vi "get_length.vi"(8 "error in (no error)":errorcluster, 11 "SpaceVector in":refnum<class "SpaceVector.lvclass">) -> (0 "error out":errorcluster, 2 "length":dbl[unit], 3 "SpaceVector out":refnum<class "SpaceVector.lvclass">)   [LabVIEW 2010, in "SpaceVector.lvclass"]
uses:
  SpaceVector.lvclass
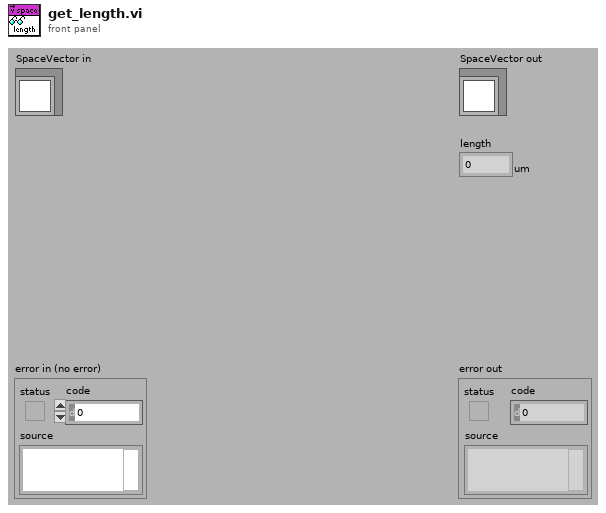
[diagram p1: front panel]
types:
  T1 = typedef "space_vector_array.ctl" = dbl[unit][]
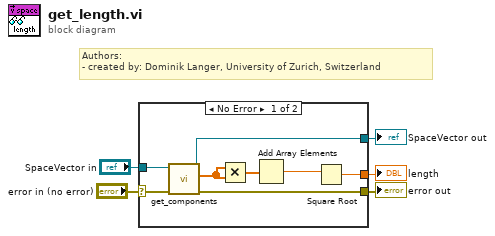
[diagram p0: block diagram]
diagram:
  # "Authors: \n- created by: Dominik Langer, University of Zurich, Switzerland"
  n1 = case shown="No Error" "error in (no error)" {
    selector: "error in (no error)" -> [w13 w15]
    tunnel: [w12 w15] -> w4
    tunnel: [w10 w14] -> w2
    tunnel: "SpaceVector in" -> [w11 w14]
    tunnel: [w6 _] -> w1
    frame No Error {
      n2 = call "get_components.vi"("error in (no error)"=w13, "SpaceVector in"=w11) -> ("error out"=w12:errorcluster, "x/y/z"=w9:T1, "SpaceVector out"=w10:refnum<class "SpaceVector.lvclass">)  [unwired: 4 in, 3 out]
      n3 = Multiply(x=w9, y=w9) -> (x*y=w8:dbl[unit][])
      n4 = Add Array Elements(numeric array=w8) -> (sum=w7:dbl[unit])
      n5 = Square Root(x=w7) -> (sqrt(x)=w6:dbl[unit])
    }
    frame Error {
    }
  }
  "error out" <- w4
  "SpaceVector out" <- w2
  "length" <- w1
